vi "Main.vi"() -> ()   [LabVIEW 2018]
doc: "Use this template to build a simple state machine design pattern. Each state executes code and determines which state to transition to."
uses:
  controls/State.ctl
  controls/Data.ctl
  <vilib>/Instr/_visa.llb/VISA Configure Serial Port (Instr).vi
panel:
  in  "LED Status":bool
  in  "LED Brightness":dbl(slide) scale=0.0..100.0
  in  "Exit":bool
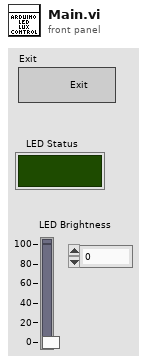
[diagram p1: front panel]
types:
  T1 = typedef "Data.ctl" = cluster{"LED Status":bool, "LED Lux":dbl}
  T2 = typedef "State.ctl" = enum16{"Initialize", "Wait for Event", "Change Brightness", "Toggle LED State", "Exit"}
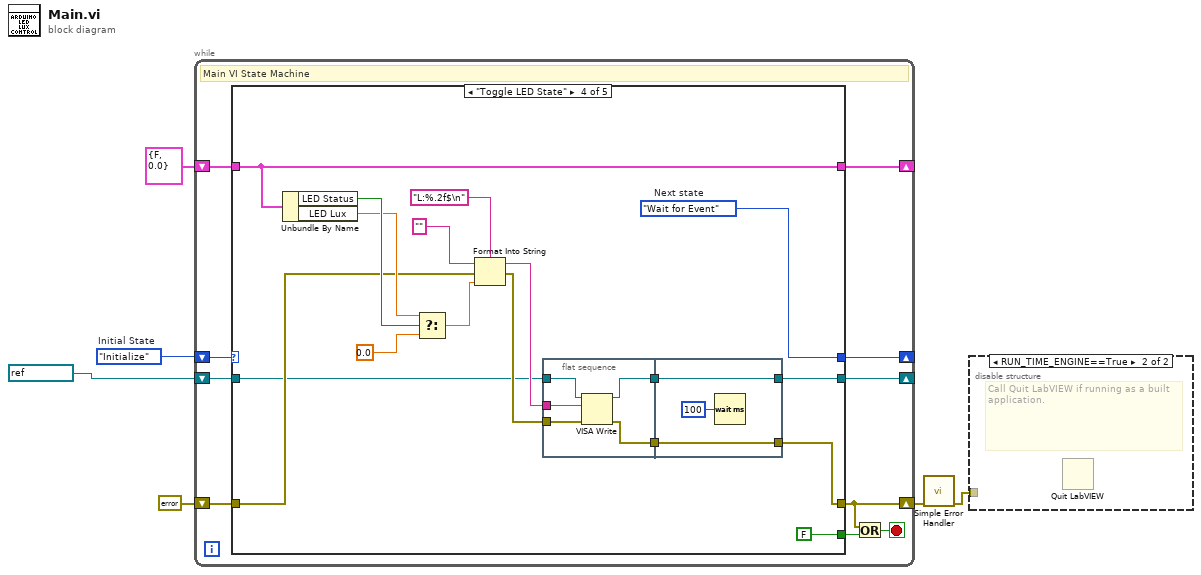
[diagram p0: block diagram]
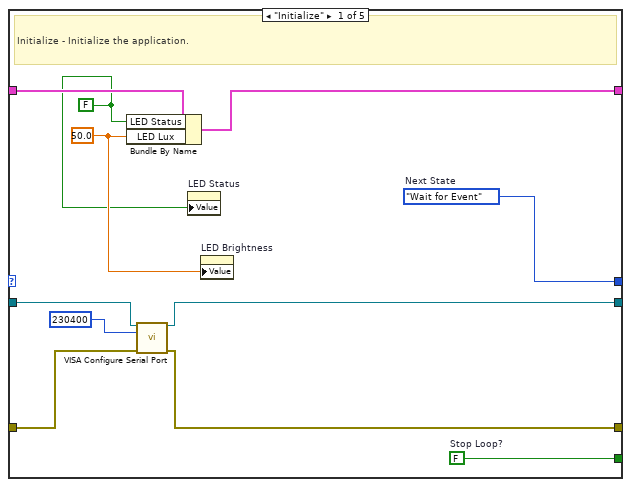
[diagram p3: hidden frame]
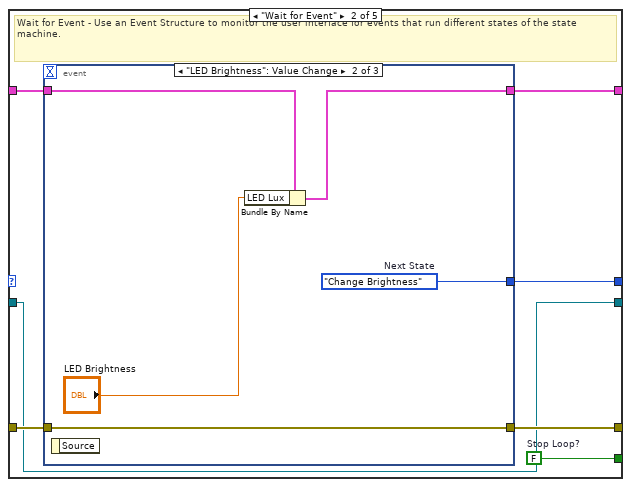
[diagram p4: hidden frame]
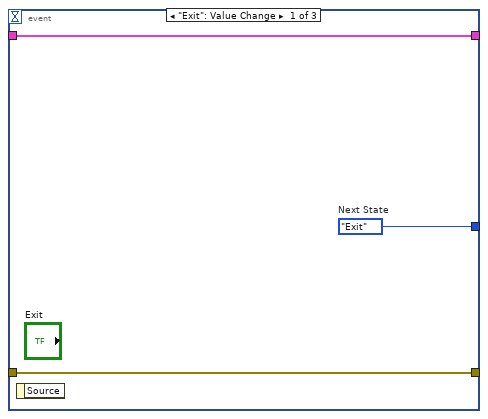
[diagram p5: hidden frame]
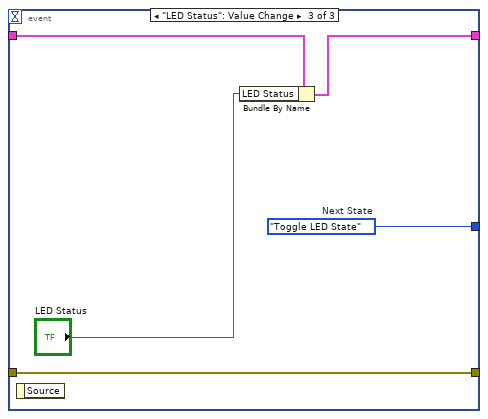
[diagram p6: hidden frame]
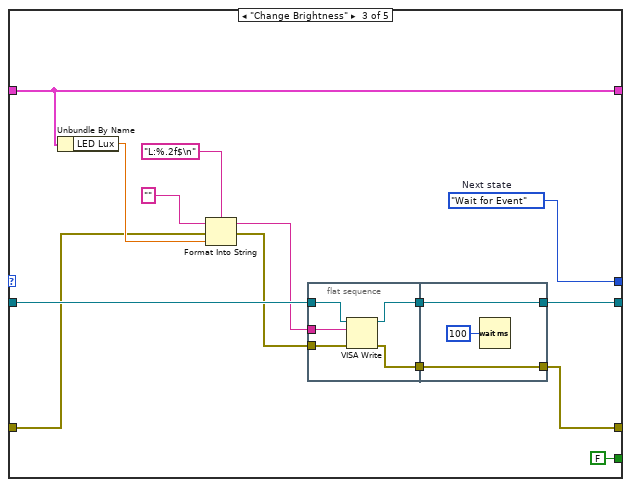
[diagram p7: hidden frame]
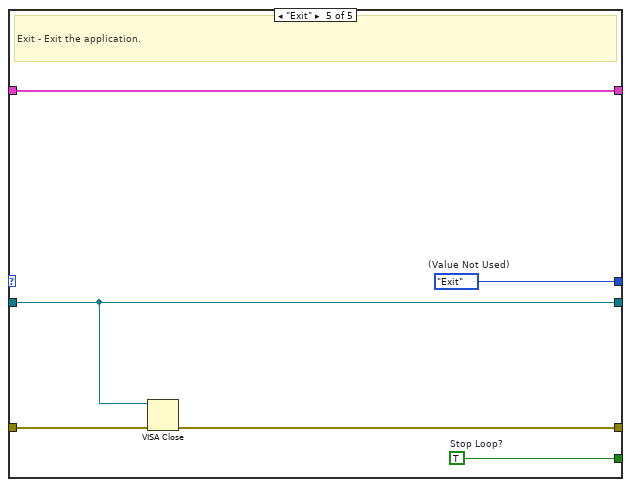
[diagram p8: hidden frame]
diagram:
  w6 = State."Initialize"  # Initial State
  n1 = while {
    shift-right: [w15] -> _
    shift-left: w6 -> [w16]
    shift-right: [w13] -> _
    shift-left: T1 {"LED Status"=FALSE, "LED Lux"=0.0} ("Data") -> [w14]
    shift-right: [w9] -> w3
    shift-left: errorcluster {"status"=FALSE, "code"=0, "source"=""} ("error constant") -> [w12]
    shift-right: [w7] -> _
    shift-left: refnum<visa-resource-name> "Arduino" ("VISA resource name") -> [w8]
    stop <- w10 stop-if-true
    # "Main VI State Machine"
    n2 = case shown="\"Toggle LED State\"" w16 {
      tunnel: [w27 w34 w57 w77 w100] -> w15
      tunnel: [w26 w33 FALSE ("Stop Loop?") FALSE ("Stop Loop?") w98] -> w11
      tunnel: w14 -> [w25 w32 w61 w86 w99]
      tunnel: [w24 w31 w61 w86 w99] -> w13
      tunnel: w12 -> [w20 w30 w53 w78 w97]
      tunnel: [w19 w29 w50 w73 w96] -> w9
      tunnel: w8 -> [w22 w28 w55 w70 w95]
      tunnel: [w18 w28 w52 w74 w95] -> w7
      frame "Initialize" {
        w23 = 50.0 ("LED Lux")
        w17 = FALSE ("LED Status")
        w26 = FALSE  # Stop Loop?
        w27 = State."Wait for Event"  # Next State
        # "Initialize - Initialize the application."
        n3 = Bundle By Name(cluster=w25, "LED Status"=w17, "LED Lux"=w23) -> (w24:T1)
        n4 = call-poly "VISA Configure Serial Port"("VISA resource name"=w22, "baud rate (9600)"=u32 230400, "error in (no error)"=w20) -> ("VISA resource name out"=w18:refnum<visa-resource-name>, "error out"=w19:errorcluster)  [unwired: 11 in]
        n5 = property on="LED Status" class="Bool (strict)"("Value"=w17) -> ()  [unwired: 2 in, 2 out]
        n6 = property on="LED Brightness" class="Slide (strict)"("Value"=w23) -> ()  [unwired: 2 in, 2 out]
      }
      frame "Wait for Event" {
        w33 = FALSE  # Stop Loop?
        # "Wait for Event - Use an Event Structure to monitor the user interface for events that run different states of the state machine."
        n7 = event shown="[1] \"LED Brightness\": Value Change" {
          selector: _ -> [_ _ _]
          dyn-events: _ -> [_ _ _]
          timeout: _ -> [_ _ _]
          tunnel: [w37 w41 w46] -> w34
          tunnel: w32 -> [w36 w40 w45]
          tunnel: [w36 w39 w44] -> w31
          tunnel: w30 -> [w35 w42 w47]
          tunnel: [w35 w42 w47] -> w29
          event "Exit": Value Change {
            w37 = State."Exit"  # Next State
            n8 = event-data() -> ()  [unwired: 1 in, 1 out]
          }
          event "LED Brightness": Value Change {
            w41 = State."Change Brightness"  # Next State
            n9 = event-data() -> ()  [unwired: 1 in, 1 out]
            n10 = Bundle By Name(cluster=w40, "LED Lux"="LED Brightness") -> (w39:T1)
          }
          event "LED Status": Value Change {
            w46 = State."Toggle LED State"  # Next State
            n11 = event-data() -> ()  [unwired: 1 in, 1 out]
            n12 = Bundle By Name(cluster=w45, "LED Status"="LED Status") -> (w44:T1)
          }
        }
      }
      frame "Change Brightness" {
        w57 = State."Wait for Event"  # Next state
        n13 = Unbundle By Name(w61) -> ("LED Lux"=w60:dbl)
        n14 = Format Into String(format string="L:%.2f$\n", initial string="", error in=w53, w60) -> (resulting string=w51:string, error out=w54:errorcluster)
        n15 = flat-sequence {
          tunnel: w55 -> [w66]
          tunnel: w54 -> [w65]
          tunnel: w51 -> [w63]
          tunnel: [w64] -> w49
          tunnel: [w62] -> w48
          tunnel: [w68] -> w50
          tunnel: [w69] -> w52
          tunnel: w49 -> [w69]
          tunnel: w48 -> [w68]
          frame #0 {
            n16 = VISA Write(VISA resource name=w66, write buffer=w63, error in (no error)=w65) -> (VISA resource name out=w64:refnum<visa-resource-name>, error out=w62:errorcluster)  [unwired: 1 out]
          }
          frame #1 {
            n17 = Wait (ms)(milliseconds to wait=u32 100) -> ()  [unwired: 1 out]
          }
        }
      }
      frame "Toggle LED State" {
        w77 = State."Wait for Event"  # Next state
        n18 = Unbundle By Name(w86) -> ("LED Status"=w82:bool, "LED Lux"=w81:dbl)
        n19 = Select(t=w81, s=w82, f=0.0) -> (s? t:f=w80:dbl)
        n20 = Format Into String(format string="L:%.2f$\n", initial string="", error in=w78, w80) -> (resulting string=w71:string, error out=w72:errorcluster)
        n21 = flat-sequence {
          tunnel: w70 -> [w91]
          tunnel: w72 -> [w90]
          tunnel: [w89] -> w76
          tunnel: [w88] -> w75
          tunnel: w71 -> [w87]
          tunnel: [w93] -> w73
          tunnel: [w94] -> w74
          tunnel: w76 -> [w94]
          tunnel: w75 -> [w93]
          frame #0 {
            n22 = VISA Write(VISA resource name=w91, write buffer=w87, error in (no error)=w90) -> (VISA resource name out=w89:refnum<visa-resource-name>, error out=w88:errorcluster)  [unwired: 1 out]
          }
          frame #1 {
            n23 = Wait (ms)(milliseconds to wait=u32 100) -> ()  [unwired: 1 out]
          }
        }
      }
      frame "Exit" {
        w98 = TRUE  # Stop Loop?
        w100 = State."Exit"  # (Value Not Used)
        # "Exit - Exit the application."
        n24 = VISA Close(VISA resource name=w95, error in (no error)=w97) -> (error out=w96:errorcluster)
      }
    }
    n25 = Or(x=w9, y=w11) -> (x .or. y?=w10:bool)
  }
  n26 = call <vilib>:"Simple Error Handler.vi"("error in (no error)"=w3) -> ("error out"=w2:errorcluster)  [unwired: 4 in, 4 out]
  n27 = disable-structure shown="RUN_TIME_ENGINE==True" {
    disable-tunnel: w2 -> [_ _]
    frame condition #0 (active) {
    }
    frame condition #1 {
      # "Call Quit LabVIEW if running as a built application."
      n28 = Quit LabVIEW() -> ()  [unwired: 1 in]
    }
  }
